vi "ring_buoy_ring.vi"(8 "error in (no error)":errorcluster, 11 "Image":T2) -> (0 "error out":errorcluster, 2 "Circles Data":T1(array[cluster]), 3 "Image Out":T2(plugin-control))   [LabVIEW 2009]
uses:
  <vilib>/vision/Image Controls.llb/IMAQ Image.ctl
  <vilib>/vision/NI_Vision_Development_Module.lvlib
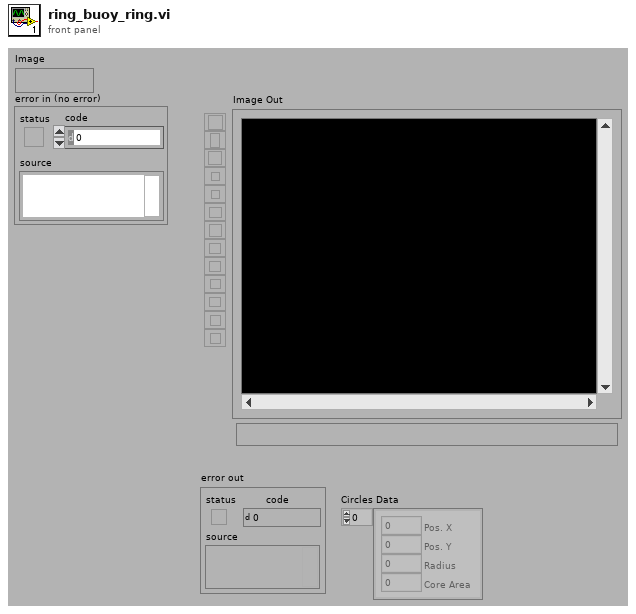
[diagram p1: front panel]
types:
  T1 = cluster{"Pos. X":i32, "Pos. Y":i32, "Radius":i32, "Core Area":i32}[]
  T2 = typedef "IMAQ Image.ctl" = refnum<image>
  T3 = cluster{"Measurement Parameter":i32, "Range Lower Value":dbl, "Range Upper Value":dbl, "Range":bool, "Measurement Type":bool}[]
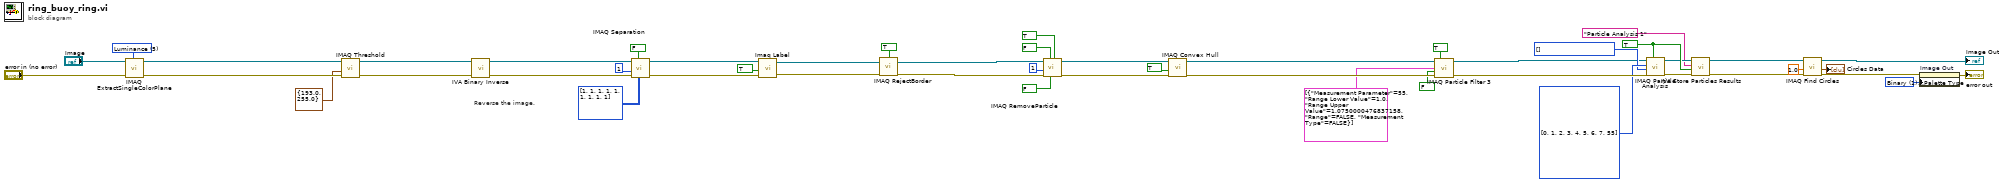
[diagram p0: block diagram]
diagram:
  w10 = u32 1 items=["Grayscale", "Binary", "Gradient", "Rainbow", "Temperature", "User Defined"] ("Palette")
  w16 = i32[] [] items=["Center of Mass X", "Center of Mass Y", "First Pixel X", "First Pixel Y", "Bounding Rect Left", "Bounding Rect Top", "Bounding Rect Right", "Bounding Rect Bottom", "Max Feret Diameter Start X", "Max Feret Diameter Start Y", "Max Feret Diameter End X", "Max Feret Diameter End Y", "Max Horiz. Segment Length Left", "Max Horiz. Segment Length Right", "Max Horiz. Segment Length Row", "-", "Bounding Rect Width", "Bounding Rect Height", "Bounding Rect Diagonal", "Perimeter", "Convex Hull Perimeter", "Holes' Perimeter", "Max Feret Diameter", "Equivalent Ellipse Major Axis", "Equivalent Ellipse Minor Axis", "Equivalent Ellipse Minor Axis (Feret)", "Equivalent Rect Long Side", "Equivalent Rect Short Side", "Equivalent Rect Diagonal", "Equivalent Rect Short Side (Feret)", "Average Horiz. Segment Length", "Average Vert. Segment Length", "Hydraulic Radius", "Waddel Disk Diameter", "-", "Area", "Holes' Area", "Particle & Holes' Area", "Convex Hull Area", "Image Area", "-", "Number of Holes", "Number of Horiz. Segments", "Number of Vert. Segments", "-", "Orientation", "Max Feret Diameter Orientation", "-", "% Area/Image Area", "% Area/(Particle & Holes' Area)", "Ratio of Equivalent Ellipse Axes", "Ratio of Equivalent Rect Sides", "-", "Elongation Factor", "Compactness Factor", "Heywood Circularity Factor", "Type Factor", "-", "Sum X", "Sum Y", "Sum XX", "Sum XY", "Sum YY", "Sum XXX", "Sum XXY", "Sum XYY", "Sum YYY", "-", "Moment of Inertia XX", "Moment of Inertia XY", "Moment of Inertia YY", "Moment of Inertia XXX", "Moment of Inertia XXY", "Moment of Inertia XYY", "Moment of Inertia YYY", "Norm. Moment of Inertia XX", "Norm. Moment of Inertia XY", "Norm. Moment of Inertia YY", "Norm. Moment of Inertia XXX", "Norm. Moment of Inertia XXY", "Norm. Moment of Inertia XYY", "Norm. Moment of Inertia YYY", "Hu Moment 1", "Hu Moment 2", "Hu Moment 3", "Hu Moment 4", "Hu Moment 5", "Hu Moment 6", "Hu Moment 7"] ("Real-World Measurements")
  w17 = i32[] [0, 1, 2, 3, 4, 5, 6, 7, 55] items=["Center of Mass X", "Center of Mass Y", "First Pixel X", "First Pixel Y", "Bounding Rect Left", "Bounding Rect Top", "Bounding Rect Right", "Bounding Rect Bottom", "Max Feret Diameter Start X", "Max Feret Diameter Start Y", "Max Feret Diameter End X", "Max Feret Diameter End Y", "Max Horiz. Segment Length Left", "Max Horiz. Segment Length Right", "Max Horiz. Segment Length Row", "-", "Bounding Rect Width", "Bounding Rect Height", "Bounding Rect Diagonal", "Perimeter", "Convex Hull Perimeter", "Holes' Perimeter", "Max Feret Diameter", "Equivalent Ellipse Major Axis", "Equivalent Ellipse Minor Axis", "Equivalent Ellipse Minor Axis (Feret)", "Equivalent Rect Long Side", "Equivalent Rect Short Side", "Equivalent Rect Diagonal", "Equivalent Rect Short Side (Feret)", "Average Horiz. Segment Length", "Average Vert. Segment Length", "Hydraulic Radius", "Waddel Disk Diameter", "-", "Area", "Holes' Area", "Particle & Holes' Area", "Convex Hull Area", "Image Area", "-", "Number of Holes", "Number of Horiz. Segments", "Number of Vert. Segments", "-", "Orientation", "Max Feret Diameter Orientation", "-", "% Area/Image Area", "% Area/(Particle & Holes' Area)", "Ratio of Equivalent Ellipse Axes", "Ratio of Equivalent Rect Sides", "-", "Elongation Factor", "Compactness Factor", "Heywood Circularity Factor", "Type Factor", "-", "Sum X", "Sum Y", "Sum XX", "Sum XY", "Sum YY", "Sum XXX", "Sum XXY", "Sum XYY", "Sum YYY", "-", "Moment of Inertia XX", "Moment of Inertia XY", "Moment of Inertia YY", "Moment of Inertia XXX", "Moment of Inertia XXY", "Moment of Inertia XYY", "Moment of Inertia YYY", "Norm. Moment of Inertia XX", "Norm. Moment of Inertia XY", "Norm. Moment of Inertia YY", "Norm. Moment of Inertia XXX", "Norm. Moment of Inertia XXY", "Norm. Moment of Inertia XYY", "Norm. Moment of Inertia YYY", "Hu Moment 1", "Hu Moment 2", "Hu Moment 3", "Hu Moment 4", "Hu Moment 5", "Hu Moment 6", "Hu Moment 7"] ("Pixel Measurements")
  w14 = TRUE ("Connectivity 4/8 (8)")
  w49 = 5 items=["Red", "Green", "Blue", "Hue", "Saturation", "Luminance", "Value", "Intensity"] ("Color Plane")
  # "Reverse the image."
  n1 = call "IMAQ ExtractSingleColorPlane"("Color Plane"=w49, "error in (no error)"="error in (no error)", "Image Src"="Image") -> ("error out"=w48:errorcluster, "Image Dst Out"=w46:T2)  [unwired: 1 in, 6 out]
  n2 = call "IMAQ Threshold"("error in (no error)"=w48, "Range"=cluster{"Lower value":sgl, "Upper value":sgl} {"Lower value"=193.0, "Upper value"=255.0}, "Image Src"=w46) -> ("error out"=w45:errorcluster, "Image Dst Out"=w44:T2)  [unwired: 3 in, 4 out]
  n3 = call <vilib>:"IVA Binary Inverse.vi"("error in (no error)"=w45, "Image In"=w44) -> ("error out"=w43:errorcluster, "Image Out"=w39:T2)  [unwired: 8 out]
  n4 = call "IMAQ Separation"("Structuring Element"=i32[][] [[1, 1, 1], [1, 1, 1], [1, 1, 1]], "Square/Hexa (Square)"=FALSE, "error in (no error)"=w43, "Nb of Erosion"=1, "Image Src"=w39) -> ("error out"=w38:errorcluster, "Image Dst Out"=w36:T2)  [unwired: 1 in, 4 out]
  n5 = call "Imaq Label"("error in (no error)"=w38, "Connectivity 4/8 (8)"=TRUE, "Image Src"=w36) -> ("error out"=w35:errorcluster, "Image Dst Out"=w33:T2)  [unwired: 1 in, 1 out]
  n6 = call "IMAQ RejectBorder"("error in (no error)"=w35, "Image Src"=w33, "Connectivity 4/8 (8)"=TRUE) -> ("error out"=w32:errorcluster, "Image Dst Out"=w27:T2)  [unwired: 1 in, 2 out]
  n7 = call "IMAQ RemoveParticle"("Connectivity 4/8 (8)"=TRUE, "Low Pass/High Pass (Low)"=FALSE, "Square/Hexa (Square)"=FALSE, "error in (no error)"=w32, "Number of Erosion"=1, "Image Src"=w27) -> ("error out"=w26:errorcluster, "Image Dst Out"=w25:T2)  [unwired: 1 in, 3 out]
  n8 = call "IMAQ Convex Hull"("error in (no error)"=w26, "Connectivity 4/8 (8)"=TRUE, "Image Src"=w25) -> ("error out"=w23:errorcluster, "Image Dst Out"=w19:T2)  [unwired: 1 in, 6 out]
  n9 = call "IMAQ Particle Filter 3"("Image Src"=w19, "Connectivity 4/8 (8)"=TRUE, "Selection Values"=T3 [{"Measurement Parameter"=55, "Range Lower Value"=1.0, "Range Upper Value"=1.0750000476837158, "Range"=FALSE, "Measurement Type"=FALSE}], "Keep/Remove Particles (F)"=FALSE ("Keep/Remove Particles"), "error in (no error)"=w23) -> ("Image Dst Out"=w15:T2, "error out"=w20:errorcluster)  [unwired: 4 in, 5 out]
  n10 = call "IMAQ Particle Analysis"("Connectivity 4/8 (8)"=w14, "error in (no error)"=w20, "Real-World Measurements"=w16, "Pixel Measurements"=w17, "Image"=w15) -> ("error out"=w11:errorcluster, "Image Out (duplicate)"=w13:T2)  [unwired: 5 out]
  n11 = call <vilib>:"IVA Store Particles Results.vi"("error in (no error)"=w11, "Connectivity 4/8 (8)"=w14, "Step Name"="Particle Analysis 1", "Image in"=w13) -> ("error out"=w5:errorcluster, "Image dup"=w6:T2)  [unwired: 6 out]
  n12 = call "IMAQ Find Circles"("error in (no error)"=w5, "Min Radius"=sgl 1.0, "Image Src"=w6) -> ("error out"=w4:errorcluster, "Circles Data"=→"Circles Data":T1, "Image Dst Out"=→"Image Out":T2)  [unwired: 5 in, 1 out]
  n13 = property on="Image Out" class="ImageControl"(error in=w4, "Palette:Palette Type"=w10) -> (error out=→"error out":errorcluster)  [unwired: 1 in, 1 out]
